vi "Dataflow Example.vi"() -> ()   [LabVIEW 2010]
doc: "This VI demonstrates reading from and writing to a file. When this is not done in the proper order, the VI will give unexpected results."
uses:
  Type.ctl
panel:
  in  "File Entry":T2
  out "Updated Text":string
  out "Current Text":string
  in  "Save":bool
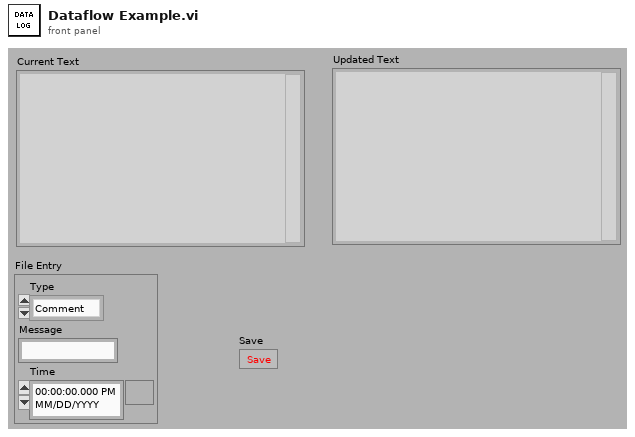
[diagram p1: front panel]
types:
  T1 = typedef "Type.ctl" = enum16{"Comment", "Question", "Concern"}
  T2 = cluster{"Type":T1, "Message":string, "Time":timestamp}
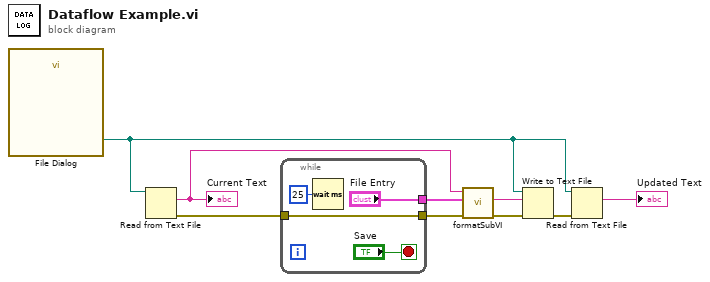
[diagram p0: block diagram]
diagram:
  n1 = call "File Dialog"() -> ("selected path"=w8:path)  [unwired: 12 in, 3 out]
  n2 = Read from Text File(file (use dialog)=w8) -> (text=w6:string, error out=w3:errorcluster)  [unwired: 3 in, 2 out]
  "Current Text" <- w6
  n3 = while {
    tunnel: ["File Entry"] -> w7
    tunnel: [w10] -> w4
    tunnel: w3 -> [w10]
    stop <- "Save" stop-if-true
    n4 = Wait (ms)(milliseconds to wait=u32 25) -> ()  [unwired: 1 out]
  }
  n5 = call "formatSubVI.vi"("error in (no error)"=w4, "Message"=w7, "Current Text"=w6) -> ("error out"=w2:errorcluster, "Text Out"=w5:string)  [unwired: 6 in, 1 out]
  n6 = Write to Text File(file (use dialog)=w8, text=w5, error in=w2) -> (error out=w1:errorcluster)  [unwired: 1 in, 2 out]
  n7 = Read from Text File(file (use dialog)=w8, error in=w1) -> (text=→"Updated Text":string)  [unwired: 2 in, 3 out]
